vi "Tom_Ben_down_sampled_trace.vi"() -> (5 "Plug in titles":string[](array[string]), 7 "Plug in values":string[](array[string]))   [LabVIEW 2010]
uses:
  Globals/Meas_global.vi
  Globals/Plug_in_data_global.vi
panel:
  in  "Post processed Results folder":path
  in  "Post processed Results folder 2":path
  in  "precision (6)":i16
  in  "Index":i32
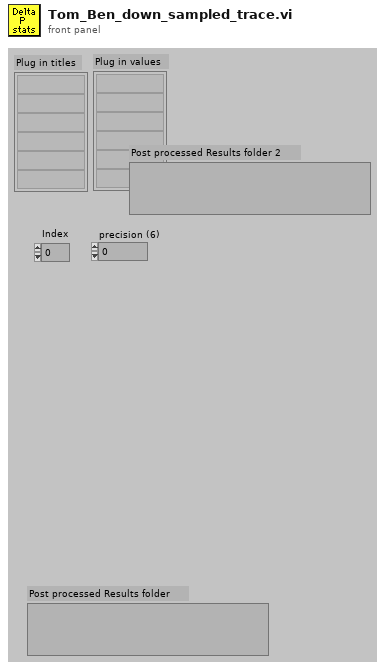
[diagram p1: front panel]
types:
  T1 = typedef "Analysis_info_cluster.ctl" = cluster{"Colour":u32, "Inst type":T2, "Inst name":string, "Symbol":string, "Code name":string, "Extra Info":string, "Inst Array":T3, "Index":i32, "Voltage Index":i32, "Extra Titles":string[], "Extra Values":string[]}
  T2 = typedef "Inst_type.ctl" = enum16{"Propeller anemometer", "Raw voltage", "Pressure Transducer", "Pitot-static tube", "Preston tube", "Hot wire", "Cross wire 1", "Cross wire 2", "Generic Linear", "Generic Polynomial", "Generic BackPoly", "Fast FID", "Thermocouple", "Cold wire", "Pulsed Wire", "LDA Vel", "LDA Tran time", "LDA Arr time"}
  T3 = typedef "Instrument_Array.ctl" = enum16{"PWA", "LDA", "Analogue"}
  T4 = enum32{"existing file", "new file", "new or existing file", "existing dir", "new dir", "new or existing dir", "existing file (use LLBs)", "new file (use LLBs)", "new or existing file (use LLBs)", "new or existing file or directory (use LLBs)"}
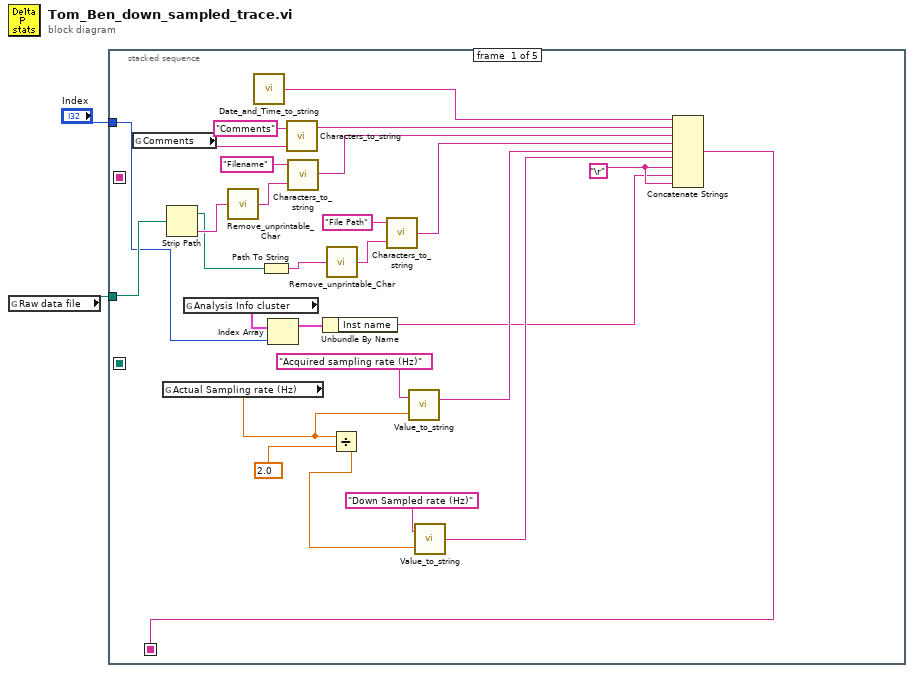
[diagram p0: block diagram]
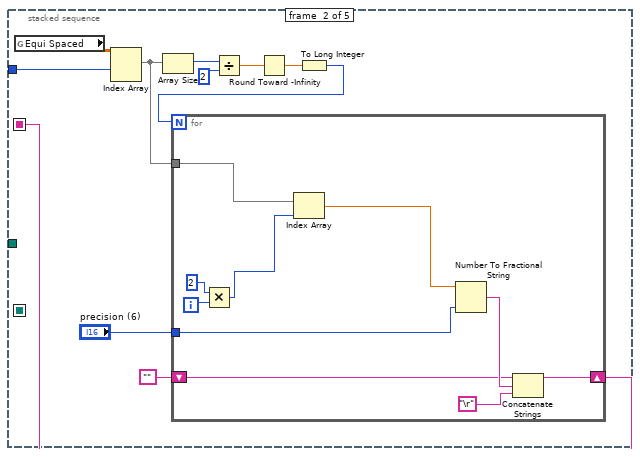
[diagram p2: hidden frame]
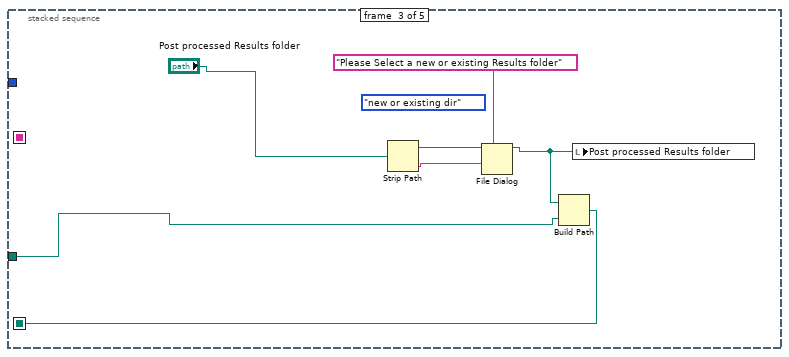
[diagram p3: hidden frame]
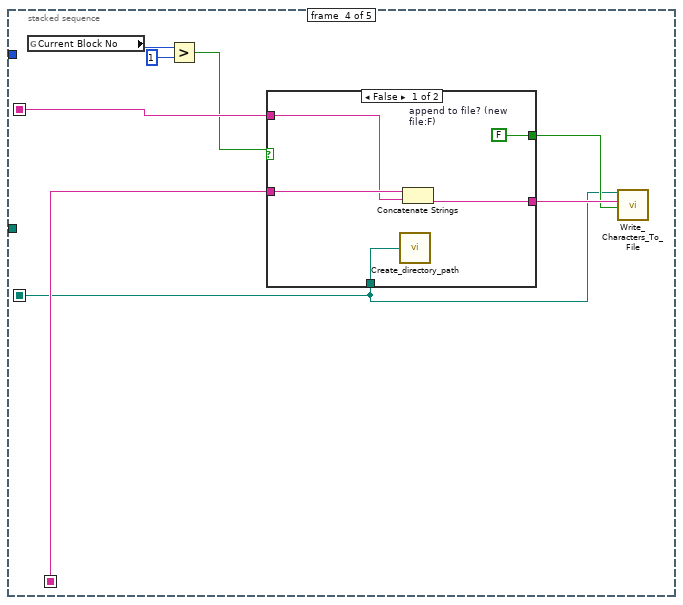
[diagram p4: hidden frame]
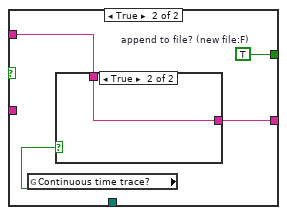
[diagram p5: hidden frame]
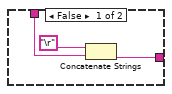
[diagram p6: hidden frame]
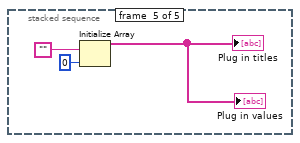
[diagram p7: hidden frame]
diagram:
  n1 = global read "Meas_global.vi" "Raw data file"() -> (w2:path)
  n2 = stacked-sequence {
    seq-local: [w25 _ _ _ _] -> [_ _ _ w65 _]
    seq-local: [_ w39 _ _ _] -> [_ _ _ w63 _]
    seq-local: [_ _ w51 _ _] -> [_ _ _ w58 _]
    tunnel: w2 -> [w23 _ w52 _ _]
    tunnel: "Index" -> [w13 w37 _ _ _]
    frame #0 {
      w4 = "\r"
      n3 = global read "Meas_global.vi" "Comments"() -> (w29:string)
      n4 = global read "Meas_global.vi" "Actual Sampling rate (Hz)"() -> (w7:dbl)
      n5 = Strip Path(path=w23) -> (stripped path=w18:path, name=w22:string)
      n6 = global read "Meas_global.vi" "Analysis Info cluster"() -> (w12:T1[])
      n7 = call "Remove_unprintable_Char.vi"("Input String"=w22) -> ("Output String"=w21:string)
      n8 = call "Date_and_Time_to_string.vi"() -> ("Date and time (spreadsheet)"=w27:string)
      n9 = Path To String(path=w18) -> (string=w17:string)
      n10 = Index Array(array=w12, index=w13) -> (element=w14:T1)
      n11 = call "Characters_to_string.vi"("Characters to write"=w29, "Label for characters"="Comments") -> ("Output string"=w26:string)
      n12 = call "Characters_to_string.vi"("Characters to write"=w21, "Label for characters"="Filename") -> ("Output string"=w16:string)
      n13 = Unbundle By Name(w14) -> ("Inst name"=w3:string)
      n14 = call "Remove_unprintable_Char.vi"("Input String"=w17) -> ("Output String"=w20:string)
      n15 = Divide(x=w7, y=2.0) -> (x/y=w9:dbl)
      n16 = call "Characters_to_string.vi"("Characters to write"=w20, "Label for characters"="File Path") -> ("Output string"=w15:string)
      n17 = call "Value_to_string.vi"("Value"=w7, "Label for value"="Acquired sampling rate (Hz)" ("Label for characters")) -> ("Output string"=w6:string)  [unwired: 1 in]
      n18 = call "Value_to_string.vi"("Value"=w9, "Label for value"="Down Sampled rate (Hz)" ("Label for characters")) -> ("Output string"=w5:string)  [unwired: 1 in]
      n19 = Concatenate Strings(w27, w26, w16, w15, w6, w5, w4, w3, w4) -> (w25:string)
    }
    frame #1 {
      n20 = global read "Plug_in_data_global.vi" "Equi Spaced"() -> (w38:dbl[][])
      n21 = Index Array(array=w38, index (row)=w37) -> (element=w34:dbl[])  [unwired: 1 in]
      n22 = Array Size(array=w34) -> (size(s)=w36:i32)
      n23 = Divide(x=w36, y=2) -> (x/y=w35:dbl)
      n24 = Round Toward -Infinity(1:w35) -> (0:w33:dbl)
      n25 = To Long Integer(number=w33) -> (32bit integer=w32:i32)
      n26 = for {
        N: w32 -> [_]
        shift-right: [w50] -> w39
        shift-left: "" -> [w43]
        tunnel: w34 -> [w45]
        tunnel: "precision (6)" -> [w42]
        i -> [w48]
        n27 = Multiply(x=2, y=w48) -> (x*y=w46:i32)
        n28 = Index Array(array=w45, index=w46) -> (element=w41:dbl)
        n29 = Number To Fractional String(number=w41, precision (6)=w42) -> (F-format string=w44:string)  [unwired: 2 in]
        n30 = Concatenate Strings(w43, w44, "\r") -> (w50:string)
      }
    }
    frame #2 {
      (unwired) T4."new or existing dir" ("select mode (2)")
      n31 = Strip Path(path="Post processed Results folder") -> (stripped path=w56:path, name=w57:string)
      n32 = File Dialog(7:"Please Select a new or existing Results folder" ("prompt"), 9:w57, 11:w56) -> (3:w53:path)  [unwired: 4 in, 3 out]
      n33 = Build Path(base path=w53, name or relative path=w52) -> (appended path=w51:path)
      n34 = local write "Post processed Results folder"(w53) -> ()
    }
    frame #3 {
      n35 = global read "Meas_global.vi" "Current Block No"() -> (w62:i32)
      n36 = Greater?(x=w62, y=1) -> (0:w60:bool)
      n37 = case shown="False" w60 {
        tunnel: w65 -> [w70 _]
        tunnel: [w69 w74] -> w64
        tunnel: w63 -> [w68 w73]
        tunnel: [w67 w72] -> w59
        tunnel: w58 -> [w66 _]
        frame False {
          w67 = FALSE  # append to file? (new file:F)
          n38 = call "Create_directory_path.vi"("Path name"=w66) -> ()  [unwired: 1 out]
          n39 = Concatenate Strings(w70, w68) -> (w69:string)
        }
        frame True {
          w72 = TRUE  # append to file? (new file:F)
          n40 = global read "Meas_global.vi" "Continuous time trace?"() -> (w71:bool)
          n41 = case shown="True" w71 {
            tunnel: [w77 w78] -> w74
            tunnel: w73 -> [w76 w78]
            frame False {
              n42 = Concatenate Strings("\r", w76) -> (w77:string)
            }
            frame True {
            }
          }
        }
      }
      n43 = call "Write_Characters_To_File.vi"("file path (dialog if empty)"=w58, "character string"=w64, "append to file? (new file:F)"=w59) -> ()  [unwired: 5 in, 1 out]
    }
    frame #4 {
      n44 = Initialize Array("", 0) -> (→"Plug in titles" →"Plug in values":string[])
    }
  }
